vi "CreateLibrary ReturnTypeDefs.vi"(8 "error in (no error)":errorcluster, 9 "Names of Registers":T1, 10 "New Name":string, 11 "Destination Directory":path) -> (0 "error out":errorcluster, 2 "TypeDef Names":string[](array[string]), 3 "TypeDef Refs":refnum<vi>[](array[refnum]))   [LabVIEW 2010]
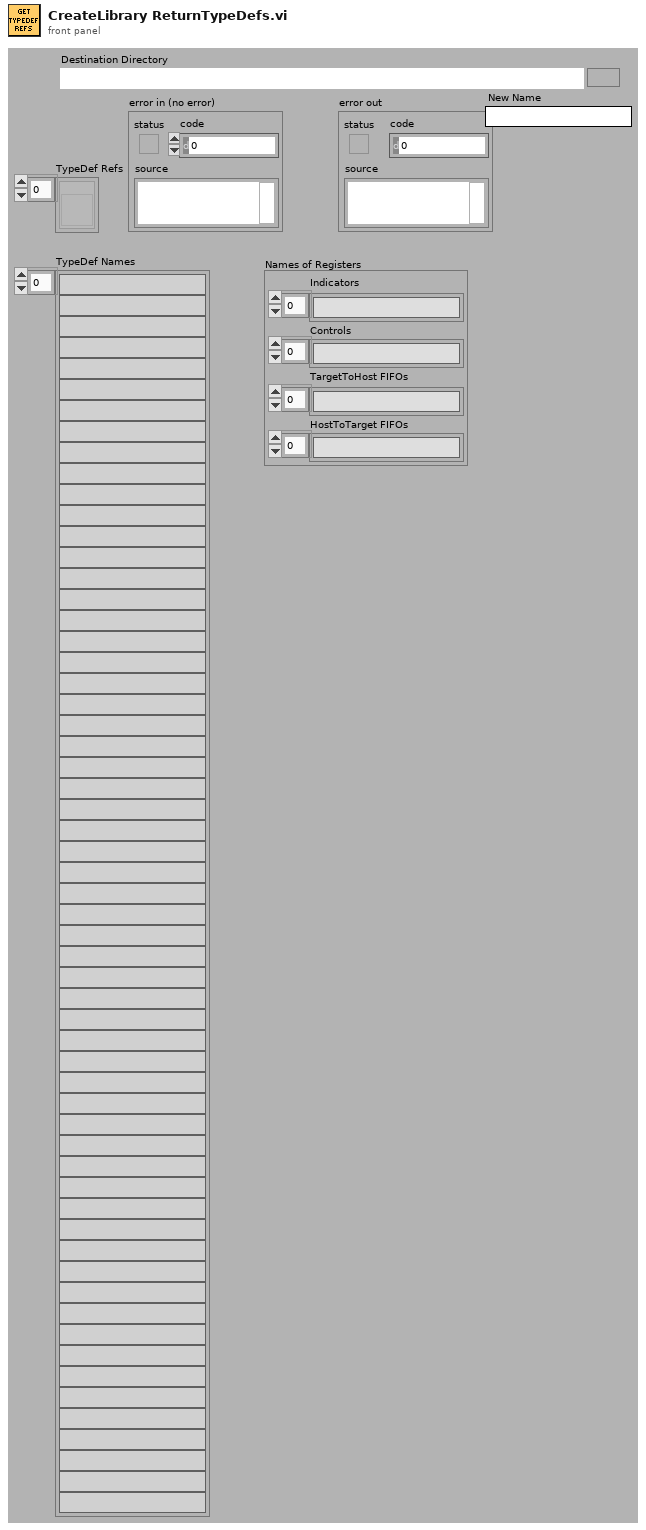
[diagram p1: front panel]
types:
  T1 = cluster{"Indicators":string[], "Controls":string[], "TargetToHost FIFOs":string[], "HostToTarget FIFOs":string[]}
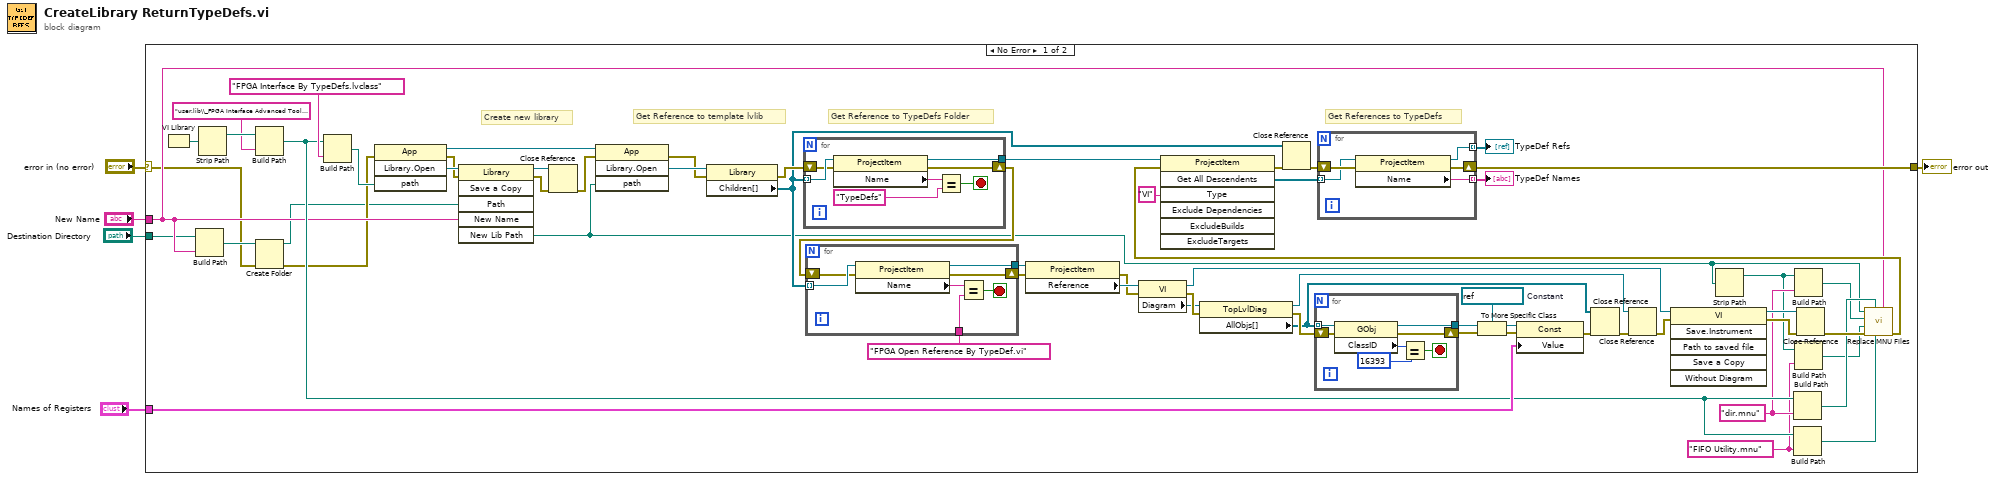
[diagram p0: block diagram]
diagram:
  n1 = case shown="No Error" "error in (no error)" {
    selector: "error in (no error)" -> [w9 w95]
    tunnel: [w62 w95] -> w5
    tunnel: "Destination Directory" -> [w7 _]
    tunnel: "New Name" -> [w11 _]
    tunnel: "Names of Registers" -> [w37 _]
    frame No Error {
      w16 = "FIFO Utility.mnu" ("name or relative path")
      w19 = "dir.mnu" ("name or relative path")
      w41 = refnum<vi> refnum  # Constant
      # "Get References to TypeDefs"
      # "Get Reference to TypeDefs Folder"
      # "Get Reference to template lvlib"
      # "Create new library"
      n2 = VI Library() -> (path=w14:path)
      n3 = Build Path(base path=w7, name or relative path=w11) -> (appended path=w10:path)
      n4 = Strip Path(path=w14) -> (stripped path=w13:path)  [unwired: 1 out]
      n5 = Build Path(base path=w13, name or relative path="user.lib\\_FPGA Interface Advanced Tools\\FPGA Interface By TypeDefs") -> (appended path=w22:path)
      n6 = Create Folder(path (use dialog)=w10, error in=w9) -> (created path=w6:path, error out=w8:errorcluster)  [unwired: 1 in, 1 out]
      n7 = Build Path(base path=w22, name or relative path="FPGA Interface By TypeDefs.lvclass") -> (appended path=w25:path)
      n8 = invoke class="App" method="Library.Open"(error in=w8, "path"=w25) -> (reference out=w57:refnum<vi>, error out=w60:errorcluster, "Open Library"=w61:refnum<vi>)  [unwired: 2 in, 1 out]
      n9 = invoke class="Library" method="Save a Copy"(reference=w61, error in=w60, "Path"=w6, "New Name"=w11) -> (reference out=w59:refnum<vi>, error out=w58:errorcluster, "New Lib Path"=w20:path)  [unwired: 2 in, 3 out]
      n10 = Close Reference(reference=w59, error in (no error)=w58) -> (error out=w56:errorcluster)
      n11 = invoke class="App" method="Library.Open"(reference=w57, error in=w56, "path"=w20) -> (error out=w54:errorcluster, "Open Library"=w55:refnum<vi>)  [unwired: 1 in, 2 out]
      n12 = property class="Library"(reference=w55, error in=w54) -> (error out=w52:errorcluster, "Children[]"=w51:refnum<vi>[])  [unwired: 1 out]
      n13 = for {
        tunnel: w51 -> [w82] mode=indexing
        tunnel: [w80] -> w63
        shift-right: [w79] -> w50
        shift-left: w52 -> [w81]
        stop <- w76 stop-if-true
        n14 = property class="ProjectItem"(reference=w82, error in=w81) -> (reference out=w80:refnum<vi>, error out=w79:errorcluster, "Name"=w77:string)
        n15 = Equal?(x=w77, y="TypeDefs") -> (x = y?=w76:bool)
      }
      n16 = for {
        tunnel: w51 -> [w75] mode=indexing
        tunnel: [w73] -> w49
        shift-right: [w72] -> w48
        shift-left: w50 -> [w74]
        tunnel: "FPGA Open Reference By TypeDef.vi" -> [w69]
        stop <- w70 stop-if-true
        n17 = property class="ProjectItem"(reference=w75, error in=w74) -> (reference out=w73:refnum<vi>, error out=w72:errorcluster, "Name"=w71:string)
        n18 = Equal?(x=w71, y=w69) -> (x = y?=w70:bool)
      }
      n19 = property class="ProjectItem"(reference=w49, error in=w48) -> (error out=w46:errorcluster, "Reference"=w47:refnum<vi>)  [unwired: 1 out]
      n20 = property class="VI"(reference=w47, error in=w46) -> (reference out=w32:refnum<vi>, error out=w45:errorcluster, "Diagram"=w44:refnum<vi>)
      n21 = property class="TopLvlDiag"(reference=w44, error in=w45) -> (reference out=w33:refnum<vi>, error out=w40:errorcluster, "AllObjs[]"=w35:refnum<vi>[])
      n22 = for {
        tunnel: w35 -> [w89] mode=indexing
        shift-right: [w84] -> w38
        shift-left: w40 -> [w85]
        tunnel: [w83] -> w39
        stop <- w86 stop-if-true
        n23 = property class="GObj"(reference=w89, error in=w85) -> (reference out=w83:refnum<vi>, error out=w84:errorcluster, "ClassID"=w88:u32)
        n24 = Equal?(x=w88, y=u32 16393) -> (x = y?=w86:bool)
      }
      n25 = To More Specific Class(target class=w41, reference=w39, error in=w38) -> (specific class reference=w42:refnum<vi>, error out=w43:errorcluster)
      n26 = property class="Const"(reference=w42, error in=w43, "Value"=w37) -> (error out=w36:errorcluster)  [unwired: 1 out]
      n27 = Close Reference(reference=w35, error in (no error)=w36) -> (error out=w34:errorcluster)
      n28 = Close Reference(reference=w33, error in (no error)=w34) -> (error out=w30:errorcluster)
      n29 = invoke class="VI" method="Save.Instrument"(reference=w32, error in=w30) -> (reference out=w31:refnum<vi>, error out=w29:errorcluster)  [unwired: 4 in, 4 out]
      n30 = Strip Path(path=w20) -> (stripped path=w17:path)  [unwired: 1 out]
      n31 = Build Path(base path=w22, name or relative path=w19) -> (appended path=w23:path)
      n32 = Build Path(base path=w22, name or relative path=w16) -> (appended path=w21:path)
      n33 = Build Path(base path=w17, name or relative path=w19) -> (appended path=w18:path)
      n34 = Build Path(base path=w17, name or relative path=w16) -> (appended path=w15:path)
      n35 = Close Reference(reference=w31, error in (no error)=w29) -> (error out=w27:errorcluster)
      n36 = call "Replace MNU Files.vi"("display name"=w11, "Palette 2 Source Path"=w21, "Palette 1 Source Path"=w23, "error in"=w27, "Palette 2 Destination Path"=w15, "Palette 1 Destination Path"=w18, "LVClass path"=w20) -> ("error out"=w26:errorcluster)  [unwired: 4 in]
      n37 = invoke class="ProjectItem" method="Get All Descendents"(reference=w63, error in=w26, "Type"="VI") -> (error out=w64:errorcluster, "All Descendents"=w65:refnum<vi>[])  [unwired: 4 in, 5 out]
      n38 = Close Reference(reference=w51, error in (no error)=w64) -> (error out=w66:errorcluster)
      n39 = for {
        tunnel: w65 -> [w93] mode=indexing
        shift-right: [w91] -> w62
        shift-left: w66 -> [w94]
        tunnel: [w92] -> w67 mode=indexing
        tunnel: [w90] -> w68 mode=indexing
        n40 = property class="ProjectItem"(reference=w93, error in=w94) -> (reference out=w90:refnum<vi>, error out=w91:errorcluster, "Name"=w92:string)
      }
      "TypeDef Names" <- w67
      "TypeDef Refs" <- w68
    }
    frame Error {
    }
  }
  "error out" <- w5
